vi "CRYCurves read & count.vi"(10 "Last curve only (F)":bool, 11 "Data file path":string) -> (0 "Curve or Result names":string[](array[string]), 1 "Canceled":bool, 2 "Data curves array":string[](array[string]), 3 "Number of curves":i32)   [LabVIEW 2013]
panel:
  out "error out":errorcluster
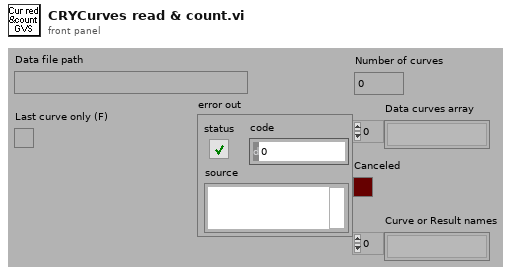
[diagram p1: front panel]
types:
  T1 = enum16{"read/write", "read-only", "write-only", "write-only (truncate)"}
  T2 = typedef "CRYResult Cluster.ctl" = cluster{"Name":string, "Margin":dbl, "unit":string, "Verdict":bool, "Limit":string, "Max/Min":string, "protected":bool, "Step No.":i32, "Test Info":string, "AutoProtect":bool}
  T3 = typedef "CRYWaveform Cluster.ctl" = cluster{"Waveform":cluster{"X0":dbl, "dX":dbl, "Y":sgl[]}, "X data":u16, "Y data":u16, "Y axis":u16, "X unit":string, "Y unit":string, "Y dB ref":dbl, "display Y":bool, "display X":bool, "Overload?":bool, "Test Info":string, "Step No.":i32, "Name":string, "protected":bool, "Sqc history":string[], "Signal Channel ID":i32, "Plot Settings":cluster{"Color":u32, "Interpolation":u8, "Point Style":u8, "Line Style":u8, "Point Color":u32, "Line Width":u8, "Bar Plot Style":u8, "Fill To":i16}, "AutoProtect":bool}
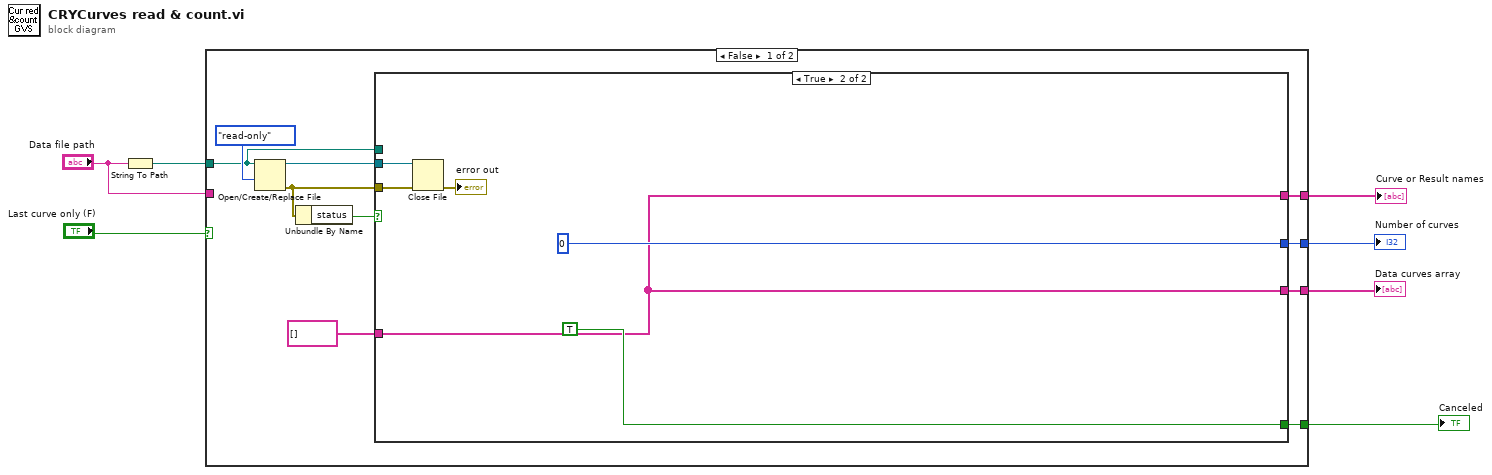
[diagram p0: block diagram]
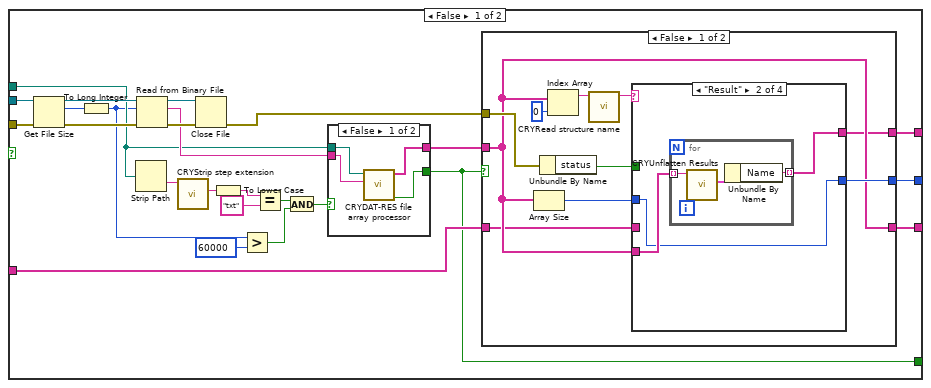
[diagram p2: hidden frame]
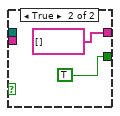
[diagram p3: hidden frame]
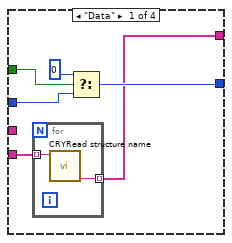
[diagram p4: hidden frame]
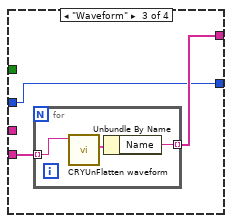
[diagram p5: hidden frame]
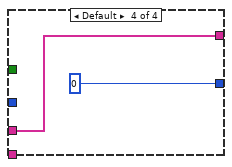
[diagram p6: hidden frame]
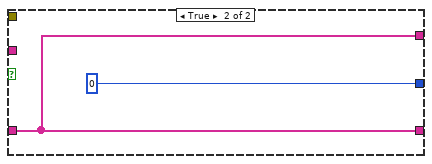
[diagram p7: hidden frame]
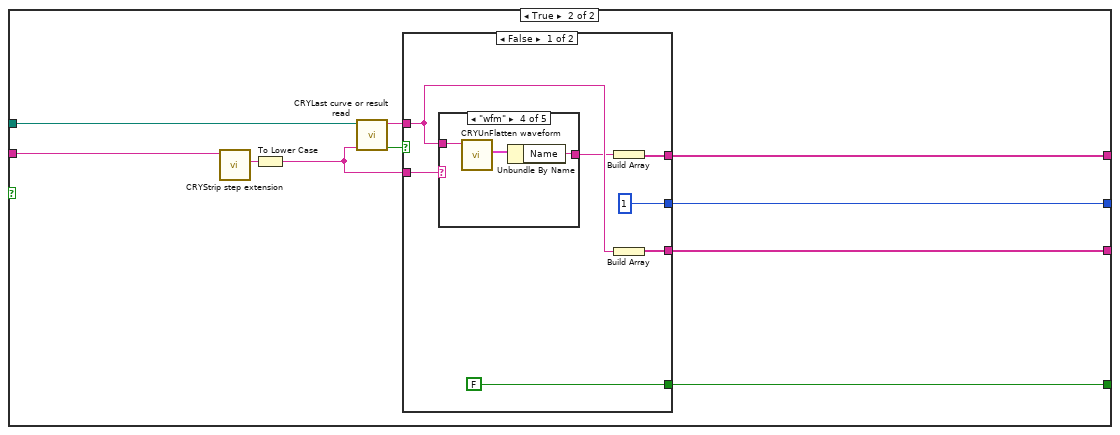
[diagram p8: hidden frame]
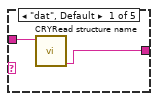
[diagram p9: hidden frame]
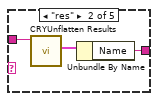
[diagram p10: hidden frame]
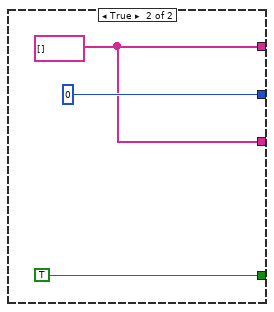
[diagram p13: hidden frame]
diagram:
  n1 = String To Path(string="Data file path") -> (path=w6:path)
  n2 = case shown="False" "Last curve only (F)" {
    tunnel: [w15 w93] -> w7
    tunnel: w6 -> [w12 w98]
    tunnel: [w10 w91] -> w5
    tunnel: [w9 w90] -> w4
    tunnel: [w8 w92] -> w3
    tunnel: "Data file path" -> [_ w97]
    frame False {
      n3 = Open/Create/Replace File(file path (use dialog)=w12, access (0:read/write)=T1."read-only" ("open mode (0)")) -> (refnum out=w13:refnum<file>, error out=w14:errorcluster)  [unwired: 1 in, 4 out]
      n4 = Unbundle By Name(w14) -> ("status"=w16:bool)
      n5 = case shown="True" w16 {
        tunnel: w14 -> [w38 w88]
        tunnel: w13 -> [w37 w87]
        tunnel: [w36 0] -> w15
        tunnel: w12 -> [w25 _]
        tunnel: string[] [] ("Data curves array") -> [w32 w84]
        tunnel: [w31 w84] -> w10
        tunnel: [w30 TRUE ("Canceled")] -> w9
        tunnel: [w29 w84] -> w8
        frame False {
          n6 = Get File Size(file=w37, error in=w38) -> (refnum out=w39:refnum<file>, size (in bytes)=w28:i64, 0:w40:errorcluster)
          n7 = To Long Integer(number=w28) -> (32bit integer=w22:i32)
          n8 = Strip Path(path=w25) -> (name=w27:string)  [unwired: 1 out]
          n9 = Read from Binary File(8:w40, 10:w22, 11:w39) -> (0:w42:errorcluster, 2:w34:string, 3:w41:refnum<file>)  [unwired: 4 out]
          n10 = call "CRYStrip step extension.vi"("Step name w/ extension"=w27) -> ("Extension (3-letter category)"=w26:string)  [unwired: 7 in, 3 out]
          n11 = Close File(refnum=w41, error in=w42) -> (error out=w35:errorcluster)  [unwired: 1 out]
          n12 = To Lower Case(string=w26) -> (all lower case string=w24:string)
          n13 = Greater?(x=w22, y=60000) -> (0:w19:bool)
          n14 = Equal?(x=w24, y="txt") -> (x = y?=w20:bool)
          n15 = And(x=w20, y=w19) -> (x .and. y?=w18:bool)
          n16 = case shown="False" w18 {
            tunnel: w34 -> [w46 _]
            tunnel: [w45 string[] [] ("Array of flat Data or Results")] -> w33
            tunnel: [w44 TRUE ("Canceled")] -> w30
            tunnel: w25 -> [w43 _]
            frame False {
              n17 = call "CRYDAT-RES file array processor.vi"("Entire file contents"=w46, "Filepath"=w43) -> ("Canceled"=w44:bool, "Array of flat Data or Results"=w45:string[])  [unwired: 8 in]
            }
            frame True {
            }
          }
          n18 = case shown="False" w30 {
            tunnel: [w56 0] -> w36
            tunnel: w35 -> [w55 _]
            tunnel: w33 -> [w51 _]
            tunnel: w32 -> [w49 w81]
            tunnel: [w51 w81] -> w31
            tunnel: [w50 w81] -> w29
            frame False {
              n19 = Array Size(array=w51) -> (size(s)=w52:i32)
              n20 = Unbundle By Name(w55) -> ("status"=w54:bool)
              n21 = Index Array(array=w51, index=0) -> (element=w57:string)
              n22 = call "CRYRead structure name.vi"("Flat data structure"=w57) -> ("Data type"=w53:string)  [unwired: 7 in, 3 out]
              n23 = case shown="\"Result\"" w53 {
                tunnel: [w61 w67 w73 0] -> w56
                tunnel: w54 -> [w64 _ _ _]
                tunnel: w52 -> [w62 w67 w73 _]
                tunnel: w51 -> [w60 w69 w75 _]
                tunnel: [w59 w68 w74 w79] -> w50
                tunnel: w49 -> [_ _ _ w79]
                frame "Data" {
                  n24 = for {
                    tunnel: w60 -> [w66] mode=indexing
                    tunnel: [w65] -> w59 mode=indexing
                    n25 = call "CRYRead structure name.vi"("Flat data structure"=w66) -> ("Curve name"=w65:string)  [unwired: 7 in, 3 out]
                  }
                  n26 = Select(t=0, s=w64, f=w62) -> (s? t:f=w61:i32)
                }
                frame "Result" {
                  n27 = for {
                    tunnel: w69 -> [w72] mode=indexing
                    tunnel: [w70] -> w68 mode=indexing
                    n28 = call "CRYUnflatten Results.vi"("Unflatten Result"=w72) -> ("Result"=w71:T2)  [unwired: 8 in, 2 out]
                    n29 = Unbundle By Name(w71) -> ("Name"=w70:string)
                  }
                }
                frame "Waveform" {
                  n30 = for {
                    tunnel: w75 -> [w78] mode=indexing
                    tunnel: [w76] -> w74 mode=indexing
                    n31 = call "CRYUnFlatten waveform.vi"("Unflatten Waveform"=w78) -> ("Waveform Cluster"=w77:T3)  [unwired: 8 in, 2 out]
                    n32 = Unbundle By Name(w77) -> ("Name"=w76:string)
                  }
                }
                frame Default {
                }
              }
            }
            frame True {
            }
          }
        }
        frame True {
          n33 = Close File(refnum=w87, error in=w88) -> (error out=→"error out":errorcluster)  [unwired: 1 out]
        }
      }
    }
    frame True {
      n34 = call "CRYStrip step extension.vi"("Step name w/ extension"=w97) -> ("Extension (3-letter category)"=w96:string)  [unwired: 7 in, 3 out]
      n35 = To Lower Case(string=w96) -> (all lower case string=w89:string)
      n36 = call "CRYLast curve or result read.vi"("Extension"=w89, "Filepath"=w98) -> ("Error"=w95:bool, "Flat Data or Result"=w94:string)  [unwired: 8 in]
      n37 = case shown="False" w95 {
        tunnel: w94 -> [w102 _]
        tunnel: [1 0] -> w93
        tunnel: [w105 w116] -> w92
        tunnel: [w104 w116] -> w91
        tunnel: [FALSE TRUE] -> w90
        tunnel: w89 -> [w101 _]
        frame False {
          n38 = case shown="\"wfm\"" w101 {
            tunnel: w102 -> [w107 w110 w111 w114 w115]
            tunnel: [w106 w108 w111 w112 w115] -> w100
            frame "dat", Default {
              n39 = call "CRYRead structure name.vi"("Flat data structure"=w107) -> ("Curve name"=w106:string)  [unwired: 7 in, 3 out]
            }
            frame "res" {
              n40 = call "CRYUnflatten Results.vi"("Unflatten Result"=w110) -> ("Result"=w109:T2)  [unwired: 8 in, 2 out]
              n41 = Unbundle By Name(w109) -> ("Name"=w108:string)
            }
            frame "txt" {
            }
            frame "wfm" {
              n42 = call "CRYUnFlatten waveform.vi"("Unflatten Waveform"=w114) -> ("Waveform Cluster"=w113:T3)  [unwired: 8 in, 2 out]
              n43 = Unbundle By Name(w113) -> ("Name"=w112:string)
            }
            frame "wav" {
            }
          }
          n44 = Build Array(w100) -> (w105:string[])
          n45 = Build Array(w102) -> (w104:string[])
        }
        frame True {
          w116 = string[] []
        }
      }
    }
  }
  "Number of curves" <- w7
  "Data curves array" <- w5
  "Canceled" <- w4
  "Curve or Result names" <- w3
